vi "output.vi"(8 "error in":errorcluster, 10 "output data":T1, 11 "DAQmx Watchdog runtime in":refnum<class "DAQmx Watchdog runtime.lvclass">) -> (0 "error out":errorcluster, 2 "output allocation":T1, 3 "DAQmx Watchdog runtime out":refnum<class "DAQmx Watchdog runtime.lvclass">)   [LabVIEW 2014, in "DAQmx Watchdog runtime.lvclass"]
doc: "Provides an interface for writing data to a module at runtime. While this interface performs no operations, a child should provide an override which may write to any open sessions, references, or interfaces."
uses:
  DAQmx Watchdog runtime.lvclass
  <vilib>/NI/Tag Bus/table/data table.ctl
  DAQmx Watchdog runtime.lvclass/DAQmx Watchdog runtime.ctl
  <vilib>/NI/Tag Bus/table/data table.lvlib
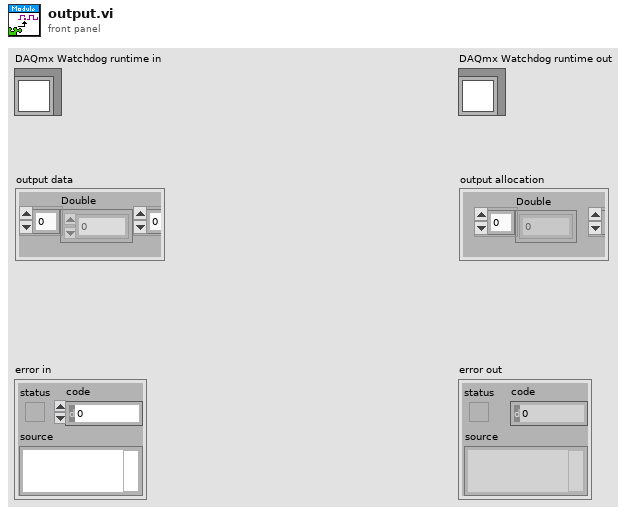
[diagram p1: front panel]
types:
  T1 = typedef "tag bus.lvlib/data table.lvlib/data table.ctl" = cluster{"Double":dbl[], "Single":sgl[], "I64":i64[], "I32":i32[], "I16":i16[], "I8":i8[], "U64":u64[], "U32":u32[], "U16":u16[], "U8":u8[], "Boolean":bool[], "String":string[], "Array of Double":cluster{"DBL Array":dbl[]}[], "Array of Single":cluster{"SGL Array":sgl[]}[], "Array of I64":cluster{"I64 Array":i64[]}[], "Array of I32":cluster{"I32 Array":i32[]}[], "Array of I16":cluster{"I16 Array":i16[]}[], "Array of I8":cluster{"I8 Array":i8[]}[], "Array of U64":cluster{"U64 Array":u64[]}[], "Array of U32":cluster{"U32 Array":u32[]}[], "Array of U16":cluster{"U16 Array":u16[]}[], "Array of U8":cluster{"U8 Array":u8[]}[], "Array of Boolean":cluster{"Boolean Array":bool[]}[], "Array of String":cluster{"String Array":string[]}[]}
  T2 = typedef "DAQmx Watchdog configuration.lvclass/output data indices.ctl" = cluster{"Boolean.Reset Timer":i32}
  T3 = typedef "DAQmx Watchdog runtime.lvclass/output user data.ctl" = cluster{"Reset Timer":bool}
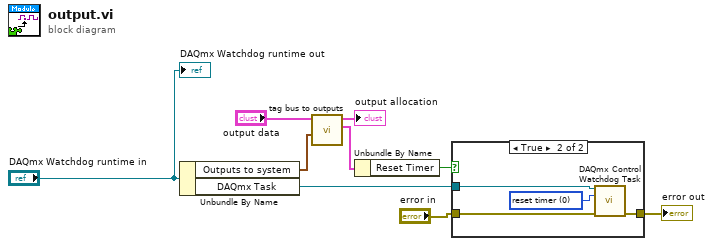
[diagram p0: block diagram]
diagram:
  n1 = Unbundle By Name("DAQmx Watchdog runtime in") -> ("Outputs to system"=w7:T2, "DAQmx Task"=w3:refnum<k21>)
  n2 = call "tag bus to outputs.vi"("indices"=w7, "tag bus in"="output data") -> ("data cluster"=w2:T3, "tag bus out"=→"output allocation":T1)  [unwired: 8 in]
  n3 = Unbundle By Name(w2) -> ("Reset Timer"=w1:bool)
  n4 = case shown="True" w1 {
    tunnel: "error in" -> [w10 w14]
    tunnel: [w10 w13] -> w4
    tunnel: w3 -> [_ w12]
    frame False {
    }
    frame True {
      w11 = 0 items=["reset timer", "clear expiration"] ("action")
      n5 = call <vilib>:"DAQmx Control Watchdog Task.vi"("task in"=w12, "action"=w11, "error in"=w14) -> ("error out"=w13:errorcluster)  [unwired: 11 in, 1 out]
    }
  }
  "error out" <- w4
  "DAQmx Watchdog runtime out" <- "DAQmx Watchdog runtime in"
